vi "p1.vi"() -> ()   [LabVIEW 2023, in "d11.lvlib"]
uses:
  d11.lvlib
  AOC/AOC.lvlib
panel:
  in  "Example":string
  in  "Example":bool
  out "Answer":i64=55944
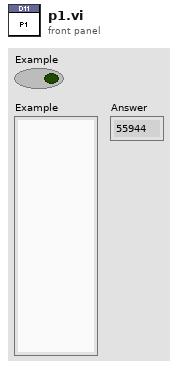
[diagram p1: front panel]
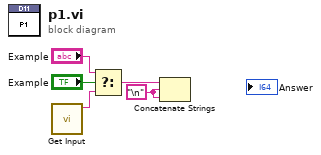
[diagram p0: block diagram]
diagram:
  w1 = "\n"
  n1 = call "Get Input.vi"() -> ("Input"=w5:string)  [unwired: 11 in]
  n2 = Select(t="Example", s="Example", f=w5) -> (s? t:f=w2:string)
  n3 = Concatenate Strings(w2, w1, w1) -> ()  [unwired: 1 out]
